vi "Initialize Mecanum Steering.vi"(8 "error in (no error)":errorcluster) -> (0 "error out":errorcluster, 3 "mecanum steering frame out":refnum<class "NI_Robotics_Mecanum Steering Frame.lvclass">)   [LabVIEW 2017]
uses:
  <vilib>/robotics/Steering/Mecanum Steering Frame/NI_Robotics_Mecanum Steering Frame.lvclass
  <vilib>/robotics/Steering/Wheel/Wheel Parameters.ctl
  <vilib>/robotics/Steering/Wheel/Rotation Direction.ctl
  Robot Parameters/Robot Parameters.vi
  <vilib>/robotics/Steering/Mecanum Wheel/Create Mecanum Wheel.vi
  <vilib>/robotics/Steering/Mecanum Steering Frame/Create Mecanum Steering Frame.vi
  <vilib>/robotics/Steering/Wheel/NI_Robotics_Wheel.lvclass
  <vilib>/robotics/Steering/Steering Frame/NI_Robotics_Steering Frame.lvclass
  <vilib>/robotics/Steering/Mecanum Wheel/NI_Robotics_Mecanum Wheel.lvclass
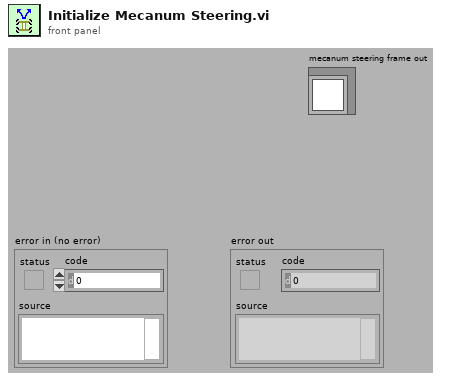
[diagram p1: front panel]
types:
  T1 = typedef "NI_Robotics_Wheel.lvclass/Wheel Parameters.ctl" = cluster{"wheel radius":dbl, "gear ratio":dbl, "forward rotation direction":T2}
  T2 = typedef "NI_Robotics_Wheel.lvclass/Rotation Direction.ctl" = u16
  T3 = cluster{"[0]":refnum<class "NI_Robotics_Mecanum Wheel.lvclass">, "[1]":refnum<class "NI_Robotics_Mecanum Wheel.lvclass">, "[2]":refnum<class "NI_Robotics_Mecanum Wheel.lvclass">, "[3]":refnum<class "NI_Robotics_Mecanum Wheel.lvclass">}
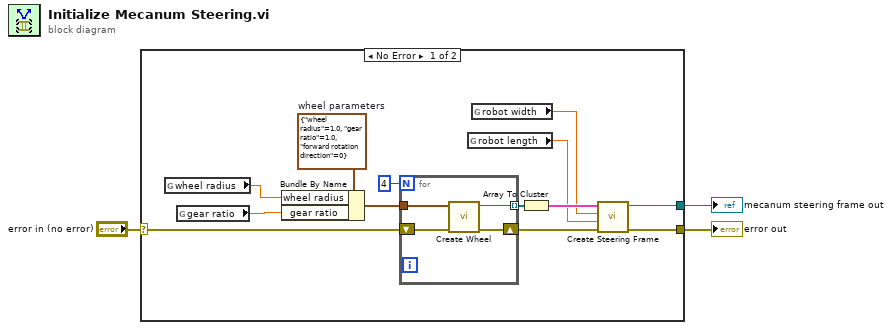
[diagram p0: block diagram]
diagram:
  n1 = case shown="No Error" "error in (no error)" {
    selector: "error in (no error)" -> [w9 w21]
    tunnel: [w11 _] -> w3
    tunnel: [w10 w21] -> w2
    frame No Error {
      w15 = T1 {"wheel radius"=1.0, "gear ratio"=1.0, "forward rotation direction"=0}  # wheel parameters
      n2 = global read "Robot Parameters.vi" "wheel radius"() -> (w7:dbl)
      n3 = global read "Robot Parameters.vi" "gear ratio"() -> (w8:dbl)
      n4 = Bundle By Name(cluster=w15, "wheel radius"=w7, "gear ratio"=w8) -> (w16:T1)
      n5 = for {
        N: 4 -> [_]
        shift-right: [w19] -> w12
        shift-left: w9 -> [w20]
        tunnel: [w18] -> w14 mode=indexing
        tunnel: w16 -> [w17]
        n6 = call-poly <vilib>:"Create Wheel.vi"("error in (no error)"=w20, "wheel parameters"=w17) -> ("error out"=w19:errorcluster, "mecanum wheel out"=w18:refnum<class "NI_Robotics_Mecanum Wheel.lvclass">)  [unwired: 8 in]
      }
      n7 = global read "Robot Parameters.vi" "robot length"() -> (w6:dbl)
      n8 = global read "Robot Parameters.vi" "robot width"() -> (w5:dbl)
      n9 = Array To Cluster(array=w14) -> (cluster=w13:T3)
      n10 = call-poly <vilib>:"Create Steering Frame.vi"("error in (no error)"=w12, "wheel separation length"=w6, "wheel separation width"=w5, "wheels"=w13) -> ("error out"=w10:errorcluster, "mecanum steering frame out"=w11:refnum<class "NI_Robotics_Mecanum Steering Frame.lvclass">)  [unwired: 6 in]
    }
    frame Error {
    }
  }
  "error out" <- w2
  "mecanum steering frame out" <- w3
